vi "IP_设置本机IP地址.vi"(8 "error in (no error)":errorcluster caption="错误输入（无错误）", 10 "IP模式":enum16{"使用特定ip", "自动获取ip"}(ring), 11 "IP Address":string) -> (0 "error out":errorcluster caption="错误输出", 2 "standard output":string caption="标准输出", 3 "标准输入":string)   [LabVIEW 2018]
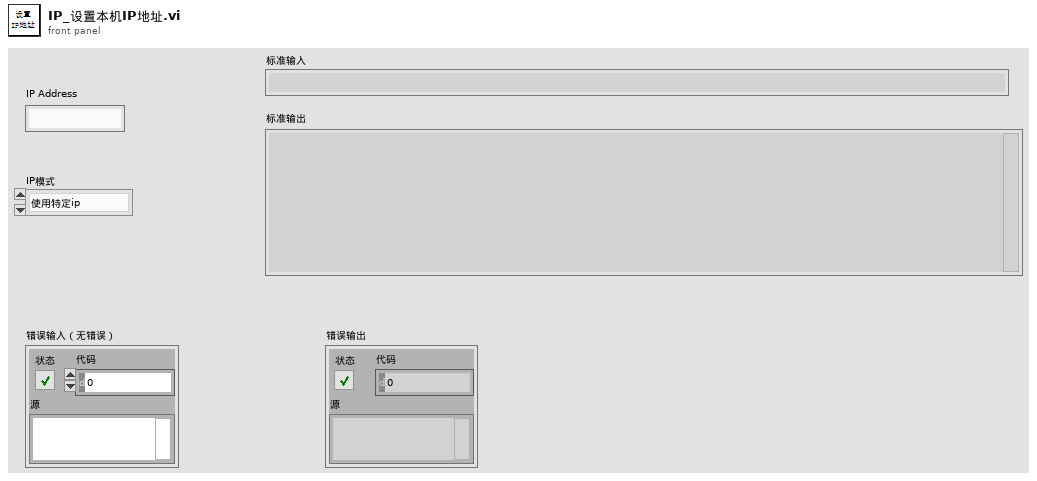
[diagram p1: front panel]
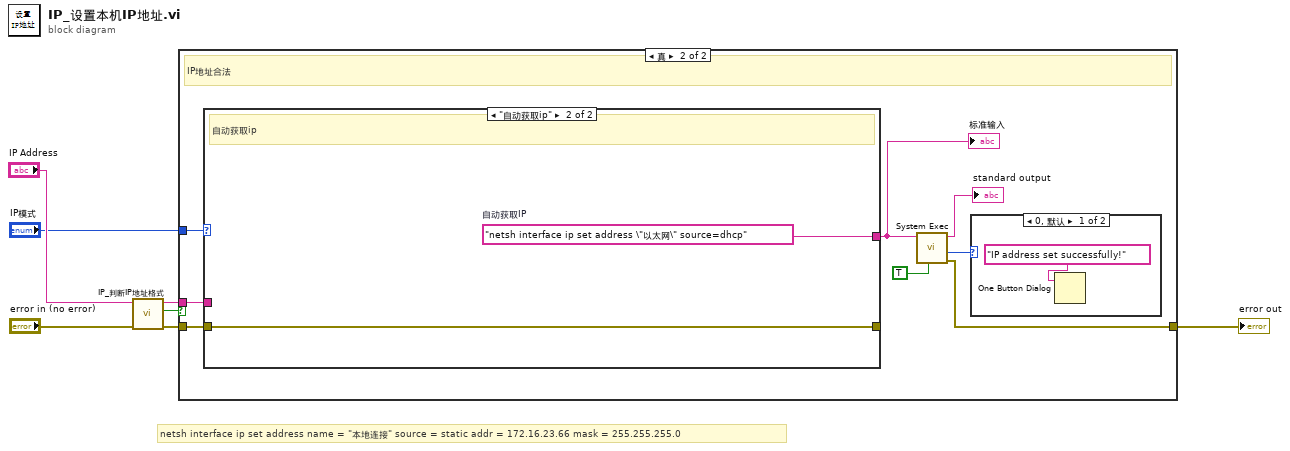
[diagram p0: block diagram]
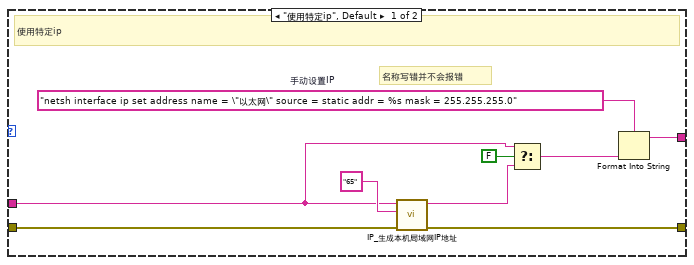
[diagram p4: hidden frame]
diagram:
  # "netsh interface ip set address name = \"本地连接\" source = static addr = 172.16.23.66 mask = 255.255.255.0"
  n1 = call "IP_判断IP地址格式.vi"("error in (no error)"="error in (no error)", "IP地址"="IP Address") -> ("error out"=w2:errorcluster, "合法IP？"=w6:bool, "IP地址 副本"=w5:string)  [unwired: 7 in]
  n2 = case shown="真" w6 {
    tunnel: w5 -> [_ w15]
    tunnel: "IP模式" -> [_ w16]
    tunnel: w2 -> [w8 w12]
    tunnel: [w8 w10] -> w1
    frame False {
      # "Invalid IP address!"
    }
    frame True {
      # "IP地址合法"
      n3 = case shown="\"自动获取ip\"" w16 {
        tunnel: w15 -> [w18 _]
        tunnel: [w25 w28] -> w14
        tunnel: w12 -> [w24 w27]
        tunnel: [w23 w27] -> _
        frame "使用特定ip", Default {
          w26 = "netsh interface ip set address name = \"以太网\" source = static addr = %s mask = 255.255.255.0"  # 手动设置IP
          # "名称写错并不会报错"
          # "使用特定ip"
          n4 = call "IP_生成本机局域网IP地址.vi"("error in (no error)"=w24, "第4段号码"="65", "IP地址"=w18) -> ("error out"=w23:errorcluster, "本机IP地址"=w19:string)  [unwired: 7 in]
          n5 = Select(t=w18, s=FALSE, f=w19) -> (s? t:f=w21:string)
          n6 = Format Into String(format string=w26, w21) -> (resulting string=w25:string)  [unwired: 2 in, 1 out]
        }
        frame "自动获取ip" {
          w28 = "netsh interface ip set address \"以太网\" source=dhcp"  # 自动获取IP
          # "自动获取ip"
        }
      }
      "标准输入" <- w14
      n7 = call <vilib>:"System Exec.vi"("run minimized? (F)"=TRUE, "command line"=w14) -> ("error out"=w10:errorcluster, "return code"=w11:i32, "standard output"=→"standard output":string)  [unwired: 6 in, 1 out]
      n8 = case shown="0, 默认" w11 {
        frame 0, Default {
          n9 = One Button Dialog(message="IP address set successfully!" ("弹出内容")) -> ()  [unwired: 1 in, 1 out]
        }
        frame 1 {
        }
      }
    }
  }
  "error out" <- w1
